vi "delate.vi"() -> ()   [LabVIEW 2018]
uses:
  <instrlib>/Delta RMC150E/Delta RMC150E.lvclass
panel:
  out "startprogram":i32[](array[numeric])
  out "实际位置":sgl(graph)
  out "实际力":sgl(graph)
  out "delateready":bool
  in  "关闭程序":bool
  in  "标定":bool
  in  "初始化":bool
  in  "急停":bool
  in  "回退":bool
  in  "长缸顶死 时间焊接":bool
  in  "长缸顶死 定位初始间隙":bool
  in  "初始间隙":i32[](array[numeric]) format="%.0x"
  in  "RampTime":i32[](array[numeric]) format="%.0x"
  in  "GapTime":i32[](array[numeric]) format="%.0x"
  in  "OpenLoopVoltage":i32[](array[numeric]) format="%.0x"
  in  "ShortMeetForce":i32[](array[numeric]) format="%.0x"
  in  "ForgeTime":i32[](array[numeric]) format="%.0x"
  in  "FrictionTime":i32[](array[numeric]) format="%.0x"
  in  "PrePressTime":i32[](array[numeric]) format="%.0x"
  in  "ForgePress":i32[](array[numeric]) format="%.0x"
  in  "FrictionPress":i32[](array[numeric]) format="%.0x"
  in  "prepress":i32[](array[numeric]) format="%.0x"
  in  "Protocol (TCP)":enum32{"TCP", "UDP"}(radio)
  in  "IP Address (rmc150.deltamotion.com)":string="rmc150.deltamotion.com"
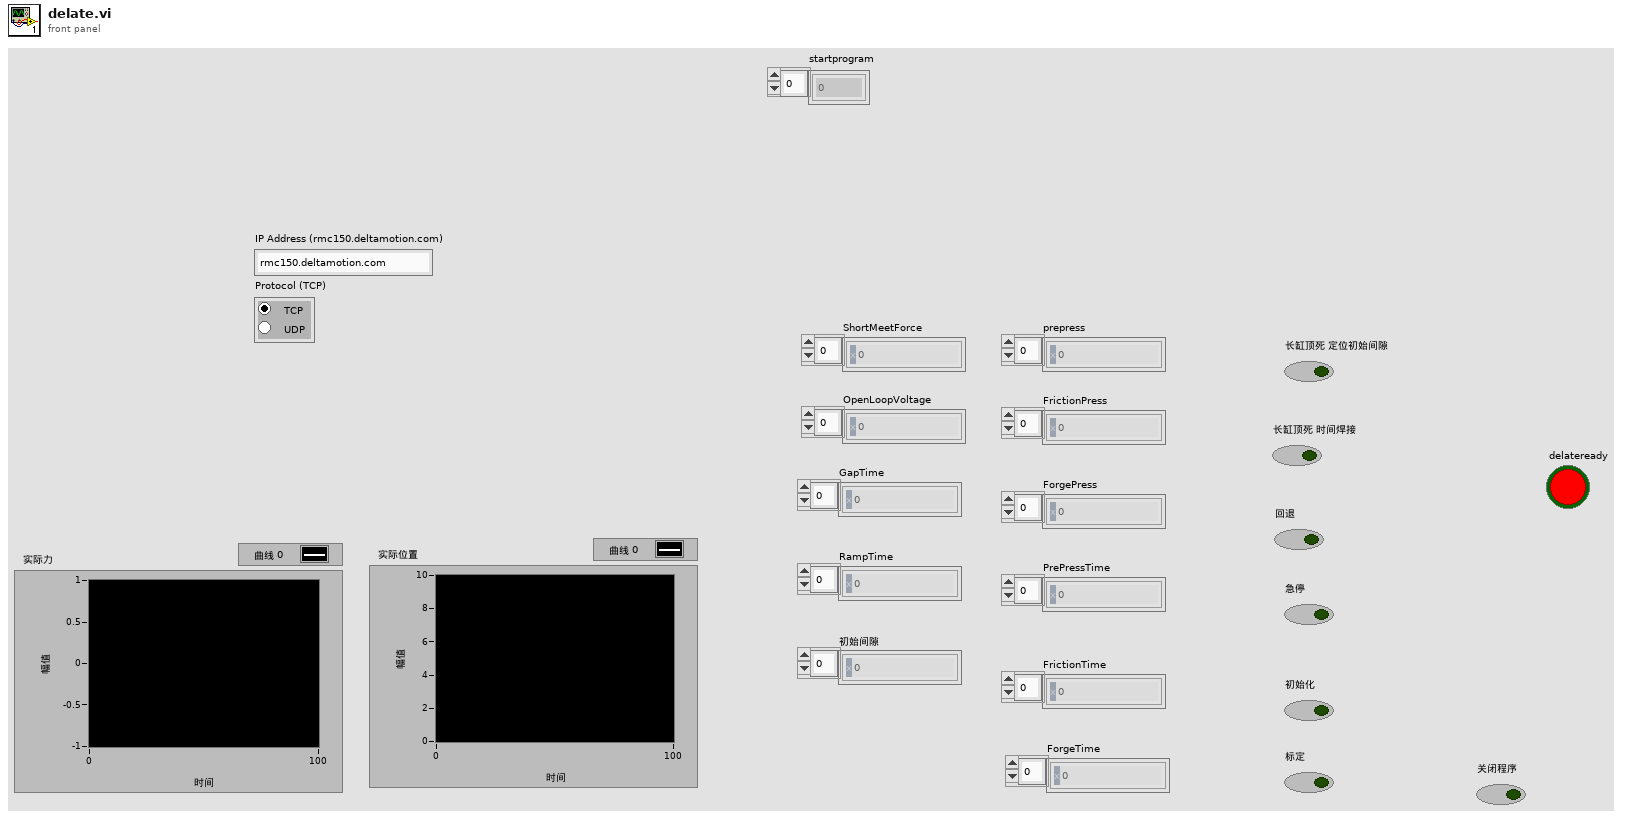
[diagram p1: front panel]
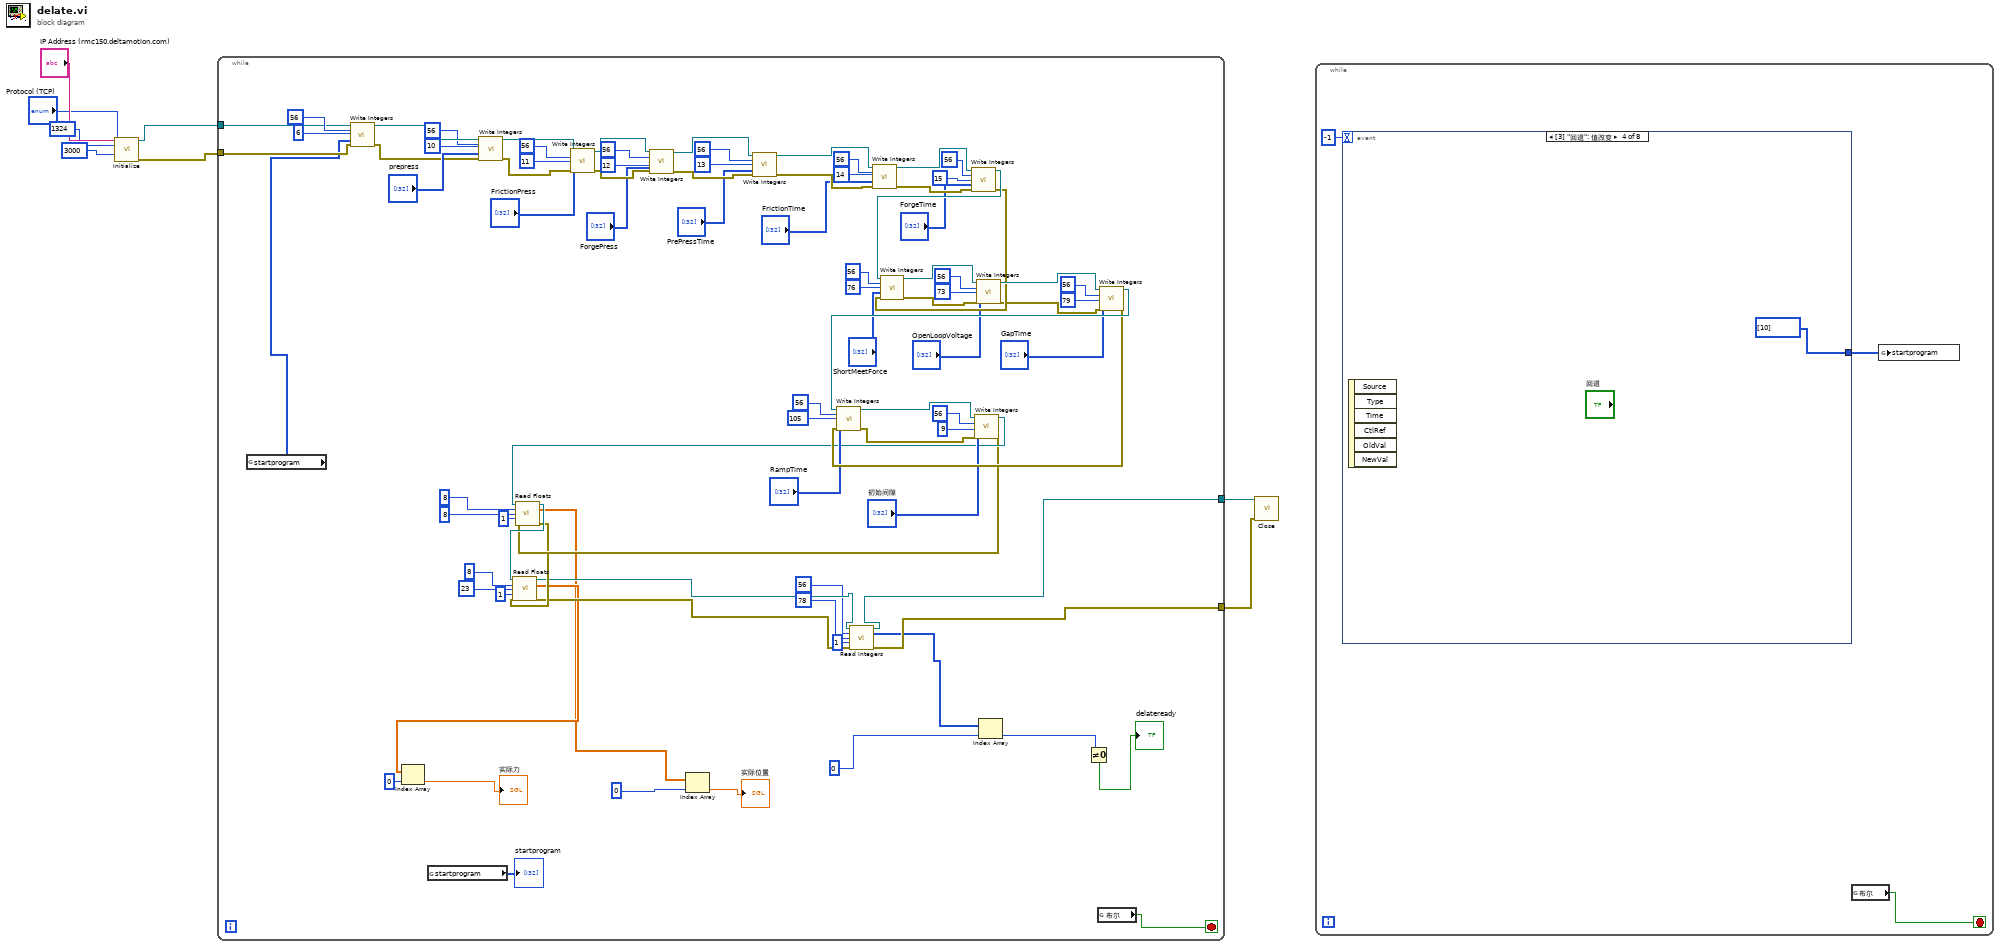
[diagram p0: block diagram]
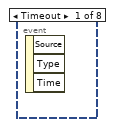
[diagram p2: hidden frame]
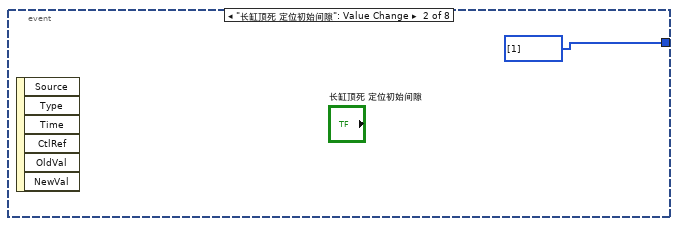
[diagram p3: hidden frame]
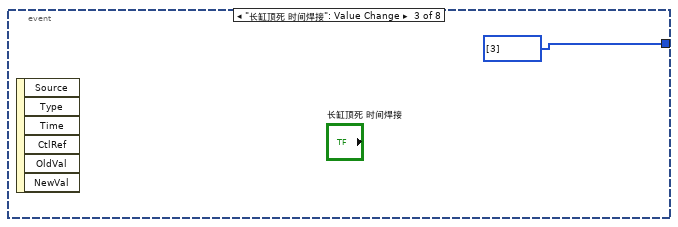
[diagram p4: hidden frame]
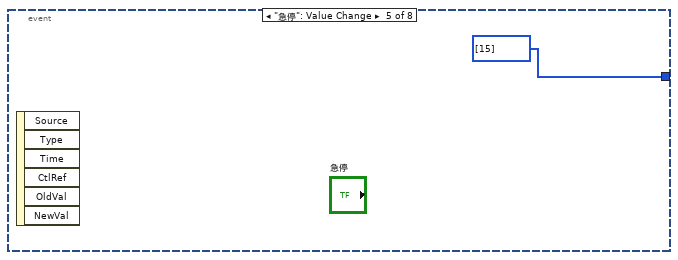
[diagram p5: hidden frame]
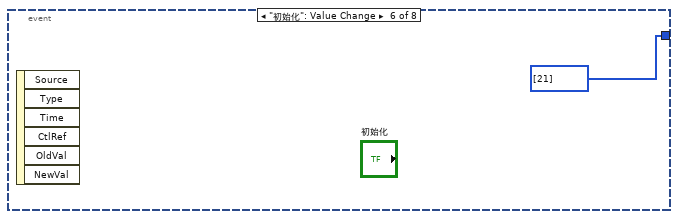
[diagram p6: hidden frame]
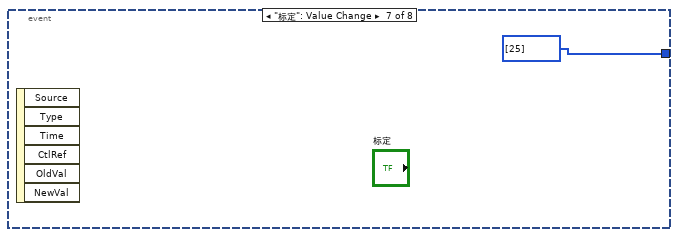
[diagram p7: hidden frame]
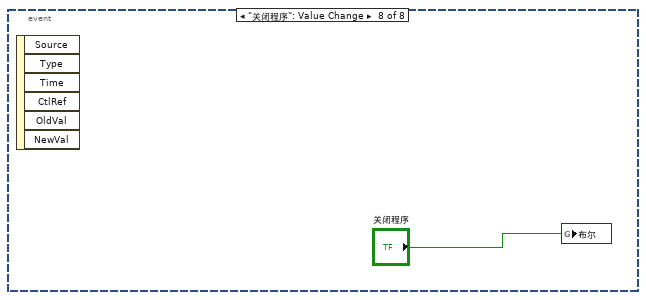
[diagram p8: hidden frame]
diagram:
  n1 = call <instrlib>:"Initialize.vi"("IP Address (rmc150.deltamotion.com)"="IP Address (rmc150.deltamotion.com)", "Port (1324)"=u16 1324, "Protocol (TCP)"="Protocol (TCP)", "Timeout (3000 ms)"=3000) -> ("RMC150E out"=w4:refnum<class "Delta RMC150E.lvclass">, "error out"=w3:errorcluster)  [unwired: 10 in]
  n2 = while {
    tunnel: w4 -> [w64]
    tunnel: w3 -> [w60]
    tunnel: [w25] -> w2
    tunnel: [w24] -> w1
    stop <- w28 stop-if-true
    n3 = global read "delate全局.vi" "startprogram"() -> (w27:i32[])
    n4 = call <instrlib>:"Write Integers.vi"("RMC150E"=w64, "File (56)"=56, "Element (0)"=6, "Data"=w27, "error in (no error)"=w60) -> ("RMC150E out"=w95:refnum<class "Delta RMC150E.lvclass">, "error out"=w59:errorcluster)  [unwired: 9 in]
    n5 = global read "delate全局.vi" "startprogram"() -> (→"startprogram":i32[])
    n6 = call <instrlib>:"Write Integers.vi"("RMC150E"=w95, "File (56)"=56, "Element (0)"=10, "Data"="prepress", "error in (no error)"=w59) -> ("RMC150E out"=w91:refnum<class "Delta RMC150E.lvclass">, "error out"=w58:errorcluster)  [unwired: 9 in]
    n7 = call <instrlib>:"Write Integers.vi"("RMC150E"=w91, "File (56)"=56, "Element (0)"=11, "Data"="FrictionPress", "error in (no error)"=w58) -> ("RMC150E out"=w72:refnum<class "Delta RMC150E.lvclass">, "error out"=w57:errorcluster)  [unwired: 9 in]
    n8 = call <instrlib>:"Write Integers.vi"("RMC150E"=w72, "File (56)"=56, "Element (0)"=12, "Data"="ForgePress", "error in (no error)"=w57) -> ("RMC150E out"=w71:refnum<class "Delta RMC150E.lvclass">, "error out"=w56:errorcluster)  [unwired: 9 in]
    n9 = call <instrlib>:"Write Integers.vi"("RMC150E"=w71, "File (56)"=56, "Element (0)"=13, "Data"="PrePressTime", "error in (no error)"=w56) -> ("RMC150E out"=w70:refnum<class "Delta RMC150E.lvclass">, "error out"=w55:errorcluster)  [unwired: 9 in]
    n10 = call <instrlib>:"Write Integers.vi"("RMC150E"=w70, "File (56)"=56, "Element (0)"=14, "Data"="FrictionTime", "error in (no error)"=w55) -> ("RMC150E out"=w69:refnum<class "Delta RMC150E.lvclass">, "error out"=w54:errorcluster)  [unwired: 9 in]
    n11 = call <instrlib>:"Write Integers.vi"("RMC150E"=w69, "File (56)"=56, "Element (0)"=15, "Data"="ForgeTime", "error in (no error)"=w54) -> ("RMC150E out"=w68:refnum<class "Delta RMC150E.lvclass">, "error out"=w53:errorcluster)  [unwired: 9 in]
    n12 = call <instrlib>:"Write Integers.vi"("RMC150E"=w68, "File (56)"=56, "Element (0)"=76, "Data"="ShortMeetForce", "error in (no error)"=w53) -> ("RMC150E out"=w67:refnum<class "Delta RMC150E.lvclass">, "error out"=w52:errorcluster)  [unwired: 9 in]
    n13 = call <instrlib>:"Write Integers.vi"("RMC150E"=w67, "File (56)"=56, "Element (0)"=73, "Data"="OpenLoopVoltage", "error in (no error)"=w52) -> ("RMC150E out"=w66:refnum<class "Delta RMC150E.lvclass">, "error out"=w51:errorcluster)  [unwired: 9 in]
    n14 = global read "delate全局.vi" "布尔"() -> (w28:bool)
    n15 = call <instrlib>:"Write Integers.vi"("RMC150E"=w66, "File (56)"=56, "Element (0)"=79, "Data"="GapTime", "error in (no error)"=w51) -> ("RMC150E out"=w65:refnum<class "Delta RMC150E.lvclass">, "error out"=w50:errorcluster)  [unwired: 9 in]
    n16 = call <instrlib>:"Write Integers.vi"("RMC150E"=w65, "File (56)"=56, "Element (0)"=105, "Data"="RampTime", "error in (no error)"=w50) -> ("RMC150E out"=w61:refnum<class "Delta RMC150E.lvclass">, "error out"=w49:errorcluster)  [unwired: 9 in]
    n17 = call <instrlib>:"Write Integers.vi"("RMC150E"=w61, "File (56)"=56, "Element (0)"=9, "Data"="初始间隙", "error in (no error)"=w49) -> ("RMC150E out"=w34:refnum<class "Delta RMC150E.lvclass">, "error out"=w32:errorcluster)  [unwired: 9 in]
    n18 = call <instrlib>:"Read Floats.vi"("RMC150E"=w34, "File (8)"=8, "Element (8)"=8, "Count (1)"=1, "error in (no error)"=w32) -> ("RMC150E out"=w33:refnum<class "Delta RMC150E.lvclass">, "Data"=w14:sgl[], "error out"=w31:errorcluster)  [unwired: 8 in]
    n19 = call <instrlib>:"Read Floats.vi"("RMC150E"=w33, "File (8)"=8, "Element (8)"=23, "Count (1)"=1, "error in (no error)"=w31) -> ("RMC150E out"=w26:refnum<class "Delta RMC150E.lvclass">, "Data"=w15:sgl[], "error out"=w23:errorcluster)  [unwired: 8 in]
    n20 = Index Array(array=w15, index=0 ("索引")) -> (element=→"实际力":sgl)
    n21 = Index Array(array=w14, index=0 ("索引")) -> (element=→"实际位置":sgl)
    n22 = call <instrlib>:"Read Integers.vi"("RMC150E"=w26, "File (56)"=56, "Element (0)"=78, "Count (1)"=1, "error in (no error)"=w23) -> ("RMC150E out"=w25:refnum<class "Delta RMC150E.lvclass">, "Data"=w18:i32[], "error out"=w24:errorcluster)  [unwired: 8 in]
    n23 = Index Array(array=w18, index=0 ("索引")) -> (element=w13:i32)
    n24 = Not Equal To 0?(x=w13) -> (x != 0?=→"delateready":bool)
  }
  n25 = call <instrlib>:"Close.vi"("RMC150E"=w2, "error in (no error)"=w1) -> ()  [unwired: 13 in, 1 out]
  n26 = while {
    stop <- w99 stop-if-true
    n27 = event shown="[3] \"回退\": 值改变" {
      selector: _ -> [_ _ _ _ _ _ _ _]
      dyn-events: _ -> [_ _ _ _ _ _ _ _]
      timeout: -1 -> [_ _ _ _ _ _ _ _]
      tunnel: [_ i32[] [1] i32[] [3] i32[] [10] i32[] [15] i32[] [21] i32[] [25] _] -> w98
      event Timeout {
        n28 = event-data() -> ()  [unwired: 1 in, 3 out]
      }
      event "长缸顶死 定位初始间隙": Value Change {
        n29 = event-data() -> ()  [unwired: 1 in, 6 out]
      }
      event "长缸顶死 时间焊接": Value Change {
        n30 = event-data() -> ()  [unwired: 1 in, 6 out]
      }
      event "回退": Value Change {
        n31 = event-data() -> ()  [unwired: 1 in, 6 out]
      }
      event "急停": Value Change {
        n32 = event-data() -> ()  [unwired: 1 in, 6 out]
      }
      event "初始化": Value Change {
        n33 = event-data() -> ()  [unwired: 1 in, 6 out]
      }
      event "标定": Value Change {
        n34 = event-data() -> ()  [unwired: 1 in, 6 out]
      }
      event "关闭程序": Value Change {
        n35 = event-data() -> ()  [unwired: 1 in, 6 out]
        n36 = global write "delate全局.vi" "布尔"("关闭程序") -> ()
      }
    }
    n37 = global read "delate全局.vi" "布尔"() -> (w99:bool)
    n38 = global write "delate全局.vi" "startprogram"(w98) -> ()
  }
